vi "LIFA_test_1.vi"() -> ()   [LabVIEW 2011]
uses:
  <vilib>/LabVIEW Interface for Arduino/LabVIEW Interface for Arduino.lvlib
panel:
  out "number":dbl
  out "Waveform Chart":dbl(graph)
  in  "stop":bool
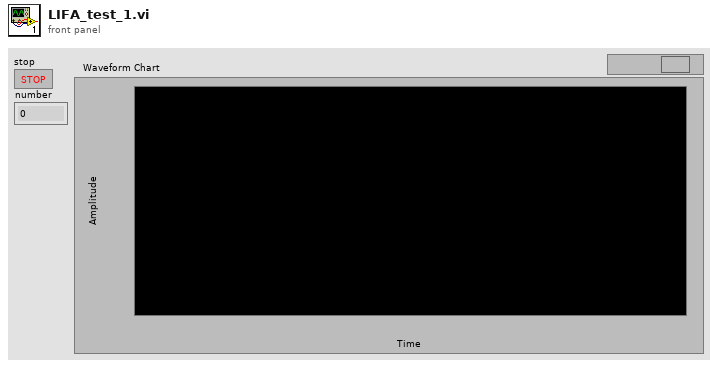
[diagram p1: front panel]
types:
  T1 = typedef "LabVIEW Interface for Arduino.lvlib/Arduino Resource.ctl" = cluster{"VISA resource":refnum<visa-resource-name>, "Board Type":T2, "Connection Type":enum8{"USB / Serial"}, "Bytes Per Packet (15)":u8}
  T2 = typedef "LabVIEW Interface for Arduino.lvlib/Board Type.ctl" = enum16{"Uno", "Mega 2560"}
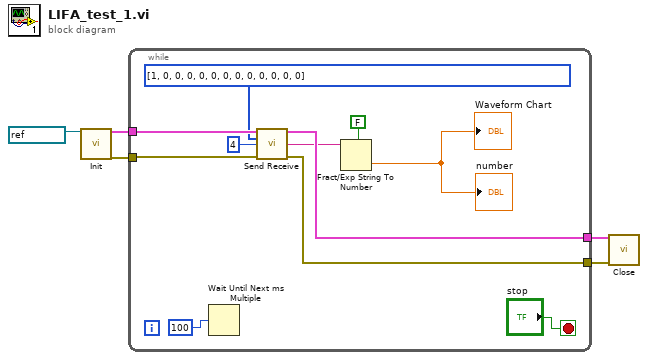
[diagram p0: block diagram]
diagram:
  n1 = call <vilib>:"Init.vi"("VISA resource"=refnum<visa-resource-name> "COM4") -> ("Arduino Resource"=w5:T1, "error out"=w4:errorcluster)  [unwired: 17 in]
  n2 = while {
    tunnel: w5 -> [w14]
    tunnel: w4 -> [w13]
    tunnel: [w12] -> w3
    tunnel: [w11] -> w2
    stop <- "stop" stop-if-true
    n3 = Wait Until Next ms Multiple(millisecond multiple=u32 100 ("millisecond timer value")) -> ()  [unwired: 1 out]
    n4 = call <vilib>:"Send Receive.vi"("Arduino Resource"=w14, "Data"=u8[] [1, 0, 0, 0, 0, 0, 0, 0, 0, 0, 0, 0, 0], "Bytes To Read (0)"=u8 4, "error in"=w13) -> ("Arduino Resource"=w12:T1, "Read Buffer"=w7:string, "error out"=w11:errorcluster)  [unwired: 9 in]
    n5 = Fract/Exp String To Number(use system decimal point (T)=FALSE, string=w7) -> (number=→"Waveform Chart" →"number":dbl)  [unwired: 2 in, 1 out]
  }
  n6 = call <vilib>:"Close.vi"("Arduino Resource"=w3, "error in"=w2) -> ()  [unwired: 13 in, 1 out]
